vi "ArcTurnLoop.vi"(8 "angle":dbl=100.0, 9 "radius":dbl=20.0, 10 "right encoder":string="My Encoder RefNum", 11 "left encoder":string="My Encoder RefNum") -> ()   [LabVIEW 2019]
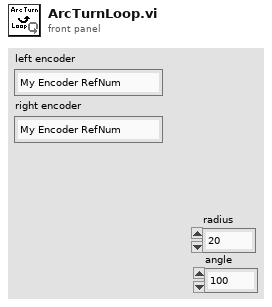
[diagram p1: front panel]
types:
  T1 = typedef "WPI_EncoderDevRef.ctl" = cluster{"DevStatus":errorcluster, "EncoderIndex":T2, "CounterIndex":T3, "DistancePerCount":dbl, "Decoding Type":T4}
  T2 = typedef "FPGA_EncoderIdx.ctl" = enum8{"Enc 0", "Enc 1", "Enc 2", "Enc 3", "Enc 4", "Enc 5", "Enc 6", "Enc 7", "Invalid"}
  T3 = typedef "FPGA_CounterCtrSystemIndex.ctl" = enum8{"Ctr 0", "Ctr 1", "Ctr 2", "Ctr 3", "Ctr 4", "Ctr 5", "Ctr 6", "Ctr 7", "Invalid"}
  T4 = typedef "WPI_EncoderType.ctl" = enum16{"1x", "2x", "4x"}
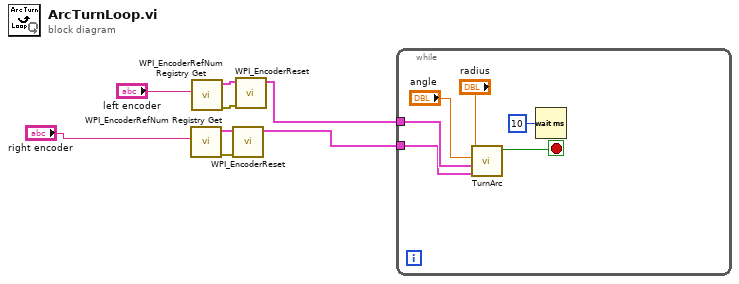
[diagram p0: block diagram]
diagram:
  n1 = call <vilib>:"WPI_EncoderRefNum Registry Get.vi"("refnum name"="right encoder") -> ("error out"=w5:errorcluster, "EncoderDevRef"=w6:T1)  [unwired: 9 in]
  n2 = call <vilib>:"WPI_EncoderRefNum Registry Get.vi"("refnum name"="left encoder") -> ("error out"=w7:errorcluster, "EncoderDevRef"=w8:T1)  [unwired: 9 in]
  n3 = call <vilib>:"WPI_EncoderReset.vi"("error in (no error)"=w5, "EncoderDevRef"=w6) -> ("EncoderDevRef"=w3:T1)  [unwired: 8 in, 1 out]
  n4 = call <vilib>:"WPI_EncoderReset.vi"("error in (no error)"=w7, "EncoderDevRef"=w8) -> ("EncoderDevRef"=w4:T1)  [unwired: 8 in, 1 out]
  n5 = while {
    tunnel: w4 -> [w13]
    tunnel: w3 -> [w12]
    stop <- w11 stop-if-true
    n6 = call "TurnArc.vi"("EncoderDevRef 2"=w12, "EncoderDevRef"=w13, "angle"="angle", "radius"="radius") -> ("stop"=w11:bool)  [unwired: 7 in]
    n7 = Wait (ms)(milliseconds to wait=u32 10) -> ()  [unwired: 1 out]
  }
